vi "Demo_ReadMovie.vi"() -> ()   [LabVIEW 2024]
doc: "Extract frames of the first the video track of any movie \nsupported by QuickTime (MOV, Mpeg, Animated Gif, Flash, AVI, etc)\n\n© Ch. Salzmann, 1994-2003"
uses:
  <userlib>/ImageProcessing/QTLIB_2595_LV86/QT_Private.ctl
  <userlib>/ImageProcessing/QTLIB_2595_LV86/QT_File.ctl
  <userlib>/ImageProcessing/QTLIB_2595_LV86/QT_FrameSelector.ctl
  <userlib>/ImageProcessing/QTLIB_2595_LV86/QT_MovieInfo.ctl
  <userlib>/ImageProcessing/QTLIB_2595_LV86/QT_Track.ctl
panel:
  out "Movie duration [s]":dbl
  out "Frame TS":i32=1800
  in  "Frame Access":T1
  out "Movie info":T2 {"Tracks"."Rate" format="%.2f"}
  in  "Access Frame ID":i32=1
  out "Picture":picture
  out "error out":errorcluster
  in  "stop":bool
  in  "Play at maximum speed":bool=TRUE
  out "Frame ID":i32=36
  in  "Path":path=path "/Chris/new Chris/Projects/QT FAT-CIN prj/FatCIN/SamplesFiles/Sample.mov"
  # "Extract frames of the first the video track of any movie supported by QuickTime (MOV, Mpeg, Animated Gif, Flash, AVI, etc)\n\n© Ch. Salzmann, 1994-2005"
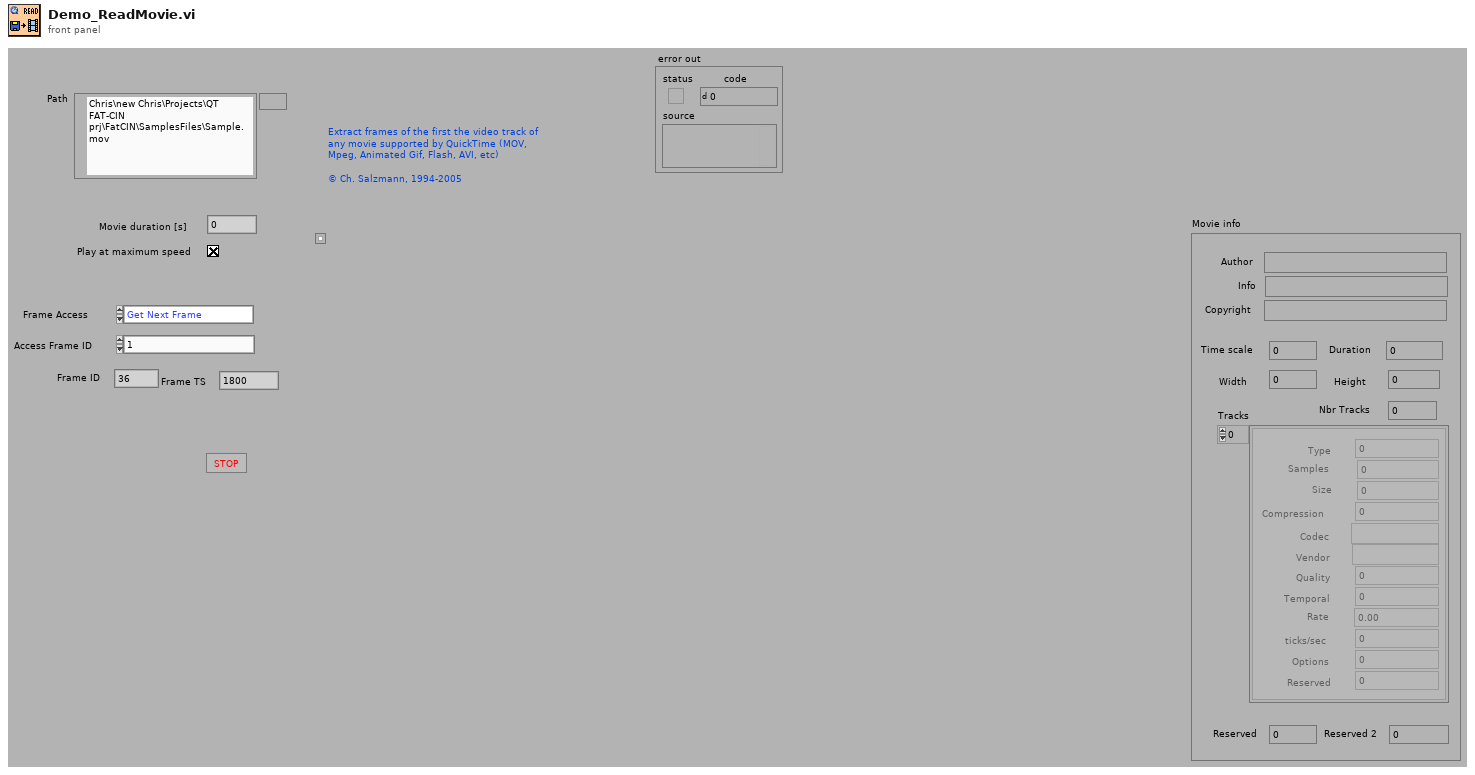
[diagram p1: front panel]
types:
  T1 = typedef "QT_FrameSelector.ctl" = enum32{"Get Next Frame", "Get Prev Frame", "Get Last Frame", "Get First Frame", "Get Frame ID", "Get Frame at Time", "reserved"}
  T2 = typedef "QT_MovieInfo.ctl" = cluster{"Author":string, "Info":string, "Copyright":string, "Time scale":i32, "Duration":i32, "Width":i32, "Height":i32, "Nbr Tracks":i32, "Tracks":T3[], "Reserved":i32, "Reserved 2":i32}
  T3 = typedef "QT_Track.ctl" = cluster{"Type":i32, "Samples":i32, "Size":i32, "Compression":i32, "Codec":string, "Vendor":string, "Quality":i32, "Temporal":i32, "Rate ":dbl, "ticks/sec":i32, "Options":i32, "Reserved":i32}
  T4 = typedef "QT_Private.ctl" = cluster{"reserved 1":i32, "reserved 2":i32, "reserved 3":i32, "reserved 4":i32}
  T5 = typedef "QT_File.ctl" = cluster{"Paths":string[], "Options":i32, "Dialogs":u32, "Reserved":i32}
  T6 = typedef "QT_Ref.ctl" = refnum<k1>
  T7 = typedef "QT_Image.ctl" = cluster{"Width":i32, "Height":i32, "Depth":i32, "data":u8[], "Compressed data":u8[], "Color table":u32[], "Duration":i32, "Options":i32, "Timestamp":i32, "ID":i32, "Reserved":i32, "Dialogs":u32}
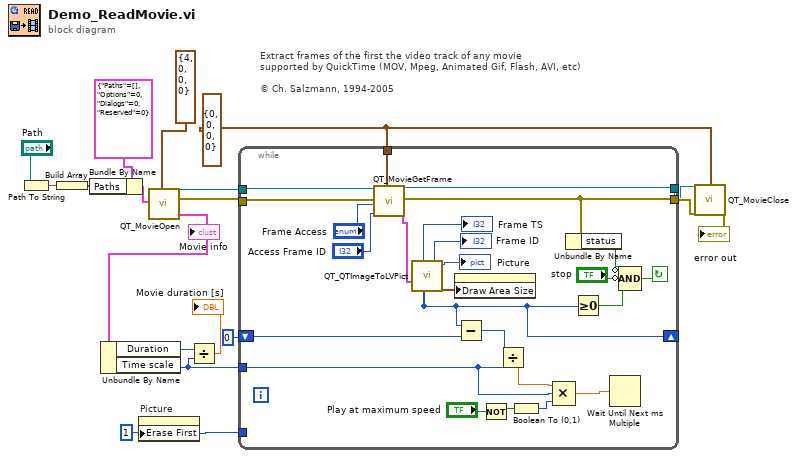
[diagram p0: block diagram]
diagram:
  w11 = u8 1 ("Erase First")
  w3 = T4 {"reserved 1"=0, "reserved 2"=0, "reserved 3"=0, "reserved 4"=0} ("Private")
  # "Extract frames of the first the video track of any movie \nsupported by QuickTime (MOV, Mpeg, Animated Gif, Flash, AVI, etc)\n\n© Ch. Salzmann, 1994-2005"
  n1 = Path To String(path="Path") -> (string=w15:string)
  n2 = Build Array(w15) -> (w7:string[])
  n3 = Bundle By Name(cluster=T5 {"Paths"=[], "Options"=0, "Dialogs"=0, "Reserved"=0} ("File Settings"), "Paths"=w7) -> (w17:T5)
  n4 = property on="Picture" class="Pict"("Erase First"=w11) -> ()  [unwired: 2 in, 2 out]
  n5 = call <userlib>:"QT_MovieOpen.vi"("File Settings"=w17, "Private"=T4 {"reserved 1"=4, "reserved 2"=0, "reserved 3"=0, "reserved 4"=0}) -> ("QT Ref Out"=w14:T6, "Movie info"=w6:T2, "error out"=w13:errorcluster)  [unwired: 1 in, 14 out]
  "Movie info" <- w6
  n6 = Unbundle By Name(w6) -> ("Duration"=w2:i32, "Time scale"=w5:i32)
  n7 = Divide(x=w2, y=w5) -> (x/y=→"Movie duration [s]":dbl)
  n8 = while {
    tunnel: w11 -> [_]
    tunnel: [w33] -> w10
    tunnel: w13 -> [w34]
    tunnel: w3 -> [w35]
    tunnel: w14 -> [w37]
    tunnel: [w36] -> w8
    shift-right: [w28] -> _
    shift-left: 0 -> [w41]
    tunnel: w5 -> [w23]
    stop <- w38 continue-if-true
    n9 = call <userlib>:"QT_MovieGetFrame.vi"("QT Ref In"=w37, "Frame Access"="Frame Access", "Frame ID"="Access Frame ID", "error in"=w34, "Private"=w35) -> ("QT Ref Out"=w36:T6, "Image Out"=w31:T7, "error out"=w33:errorcluster)  [unwired: 12 out]
    n10 = call <userlib>:"QT_QTImageToLVPict.vi"("Image/Movie Out"=w31) -> ("Timestamp"=w28:i32, "ID"=→"Frame ID":i32, "Picture color"=→"Picture":picture, "Pict Draw Area Size"=w29:cluster{"Width":i16, "Height":i16})  [unwired: 2 in, 13 out]
    "Frame TS" <- w28
    n11 = property on="Picture" class="Pict"("Draw Area Size"=w29) -> ()  [unwired: 2 in, 2 out]
    n12 = Subtract(x=w28, y=w41) -> (x-y=w40:i32)
    n13 = Not(x="Play at maximum speed") -> (.not. x?=w19:bool)
    n14 = Divide(x=w40, y=w23) -> (x/y=w39:dbl)
    n15 = Boolean To (0,1)(Boolean=w19) -> (0, 1=w20:i16)
    n16 = Compound Arithmetic op=MULTIPLY(w39, w23, w20) -> (w22:dbl)
    n17 = Unbundle By Name(w33) -> ("status"=w32:bool)
    n18 = Greater Or Equal To 0?(x=w28) -> (x >= 0?=w42:bool)
    n19 = Wait Until Next ms Multiple(millisecond multiple=w22) -> ()  [unwired: 1 out]
    n20 = Compound Arithmetic op=AND(invert w32, invert "stop", w42) -> (w38:bool)
  }
  n21 = call <userlib>:"QT_MovieClose.vi"("QT Ref In"=w8, "error in (no error)"=w10, "Private"=w3) -> ("error out"=→"error out":errorcluster)  [unwired: 16 out]
